vi "Get Result.vi"(8 "error in (no error)":errorcluster, 11 "LakeShore T Controller in":refnum<class "Mag Lab Temperature Controller.lvclass">) -> (0 "error out":errorcluster, 2 "Mag Lab Result.lvclass":refnum<class "Mag Lab Result.lvclass">, 3 "LakeShore T Controller out":refnum<class "Mag Lab Temperature Controller.lvclass">)   [LabVIEW 2015, in "Mag Lab Temperature Controller.lvclass"]
uses:
  Mag Lab Temperature Controller.lvclass
  Mag Lab Result/Mag Lab Result.lvclass
  T controller parameters.ctl
  Instruments/Neocera/Neocera Set Point Aproach.ctl
  Mag Lab Result/Payload/DBL Payload/DBL Payload.lvclass
  Mag Lab Hardware.lvclass/Mag Lab Hardware.ctl
  Mag Lab Root/Mag Lab Root.lvclass/Mag Lab Root.ctl
  Mag Lab Result/Payload/Payload.lvclass/Payload.ctl
  Mag Lab Result/Mag Lab Result.lvclass/Mag Lab Result.ctl
  Mag Lab Result/Payload/Write Name.vi
  Mag Lab Properties/Mag Lab Parameters.lvclass
  Mag Lab Hardware.lvclass
  Mag Lab Root/Mag Lab Root.lvclass
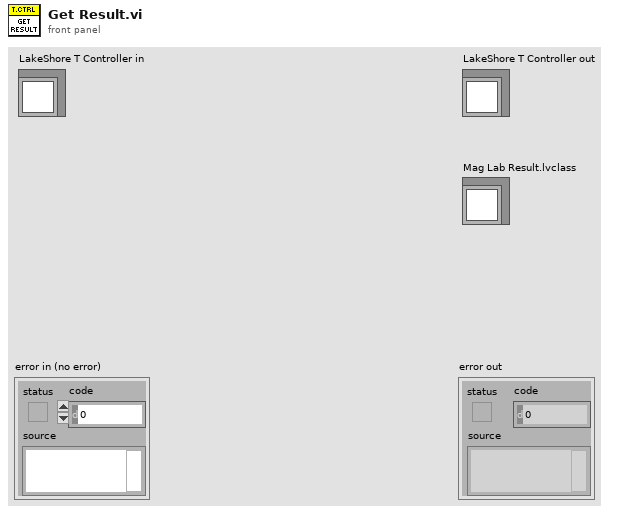
[diagram p1: front panel]
types:
  T1 = typedef "T controller parameters.ctl" = cluster{"Record heater":bool, "Record RAW":bool, "Set point":dbl, "Heater range":dbl, "Approach":T2, "Ramp rate, K/min":dbl, "Record Channels":string[], "Settling time ":dbl, "Settling range":dbl, "P":dbl, "I":dbl, "D":dbl, "Temperature Control":bool}
  T2 = typedef "Neocera Set Point Aproach.ctl" = enum16{"Instant", "Ramp"}
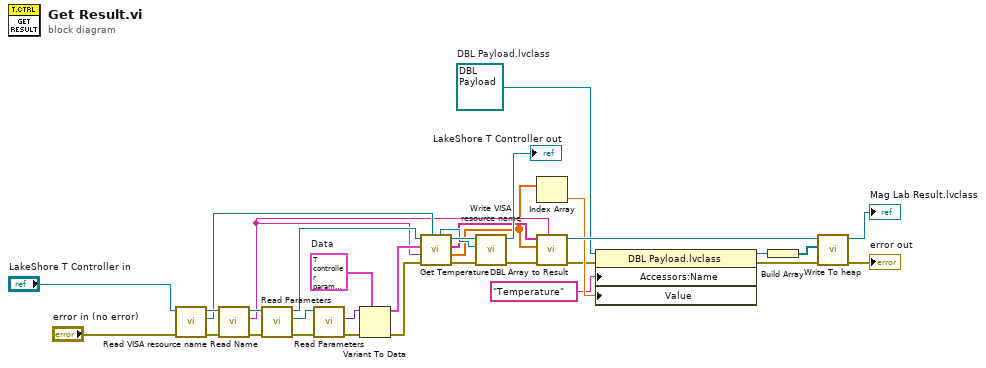
[diagram p0: block diagram]
diagram:
  w9 = refnum<class "DBL Payload.lvclass"> refnum  # DBL Payload.lvclass
  w24 = T1 {"Record heater"=FALSE, "Record RAW"=FALSE, "Set point"=0.0, "Heater range"=0.0, "Approach"=enum."Instant", "Ramp rate, K/min"=1.0, "Record Channels"=[], "Settling time "=60.0, "Settling range"=0.1, "P"=0.0, "I"=0.0, "D"=0.0, "Temperature Control"=FALSE}  # Data
  n1 = call "Read VISA resource name.vi"("error in (no error)"="error in (no error)", "Mag Lab Hardware in"="LakeShore T Controller in") -> ("error out"=w32:errorcluster, "VISA resource name"=w17:refnum<visa-resource-name>, "Mag Lab Hardware out"=w33:refnum<class "Mag Lab Temperature Controller.lvclass">)  [unwired: 7 in]
  n2 = call "Read Name.vi"("error in (no error)"=w32, "Mag Lab Root in"=w33) -> ("error out"=w26:errorcluster, "Name"=w11:string, "Mag Lab Root out"=w25:refnum<class "Mag Lab Temperature Controller.lvclass">)  [unwired: 7 in]
  n3 = call-dynamic "Read Parameters.vi"("error in (no error)"=w26, "Mag Lab Root in"=w25) -> ("error out"=w13:errorcluster, "Mag Lab Parameters.lvclass"=w23:refnum<class "Mag Lab Parameters.lvclass">, "Mag Lab Root out"=w21:refnum<class "Mag Lab Temperature Controller.lvclass">)  [unwired: 7 in]
  n4 = call-dynamic "Read Parameters.vi"("error in (no error)"=w13, "Mag Lab Parameters in"=w23) -> ("error out"=w12:errorcluster, "Parameters"=w14:variant)  [unwired: 7 in, 1 out]
  n5 = Variant To Data(error in=w12, type=w24, Variant=w14) -> (data=w15:T1, error out=w22:errorcluster)
  n6 = call-dynamic "Get Temperature.vi"("VISA resource"=w17, "error in (no error)"=w22, "Name"=w11, "Data"=w15, "Mag Lab Temperature Controller in"=w21) -> ("error out"=w19:errorcluster, "Channel data"=w8:dbl[], "Channel names"=w16:string[], "Mag Lab Temperature Controller out"=w20:refnum<class "Mag Lab Temperature Controller.lvclass">, "VISA resource out"=w18:refnum<visa-resource-name>)  [unwired: 1 in, 1 out]
  n7 = call "Write VISA resource name.vi"("error in (no error)"=w19, "VISA resource name"=w18, "Mag Lab Hardware in"=w20) -> ("error out"=w31:errorcluster, "Mag Lab Hardware out"=→"LakeShore T Controller out":refnum<class "Mag Lab Temperature Controller.lvclass">)  [unwired: 7 in]
  n8 = Index Array(array=w8) -> (element=w7:dbl)  [unwired: 1 in]
  n9 = call "DBL Array to Result.vi"("Result name"=w11, "error in (no error)"=w31, "Data"=w8, "Channel Names"=w16) -> ("error out"=w3:errorcluster, "Mag Lab Result out"=w27:refnum<class "Mag Lab Result.lvclass">)  [unwired: 6 in]
  n10 = property class="DBL Payload.lvclass"(reference=w9, error in=w3, "Accessors:Name"="Temperature" ("Name"), "Value"=w7) -> (reference out=w5:refnum<class "DBL Payload.lvclass">, error out=w2:errorcluster)
  n11 = Build Array(w5) -> (w4:refnum<class "DBL Payload.lvclass">[])
  n12 = call "Write To heap.vi"("error in (no error)"=w2, "To heap"=w4, "Mag Lab Result in"=w27) -> ("error out"=→"error out":errorcluster, "Mag Lab Result out"=→"Mag Lab Result.lvclass":refnum<class "Mag Lab Result.lvclass">)  [unwired: 7 in]
